vi "Count Up Down.vi"(6 "load":bool, 7 "reset":bool, 8 "error in":errorcluster, 9 "preset value":u32=10, 10 "count down":bool, 11 "count up":bool) -> (0 "error out":errorcluster, 1 "counter value":u32, 2 "count down done":bool, 3 "count up done":bool)   [LabVIEW 2020, in "NI_FunctionBlock Libraries.lvlib"]
uses:
  <vilib>/functionblocks/NI_FunctionBlock Libraries.lvlib
  <vilib>/ptbypt/NI_PtbyPt.lvlib
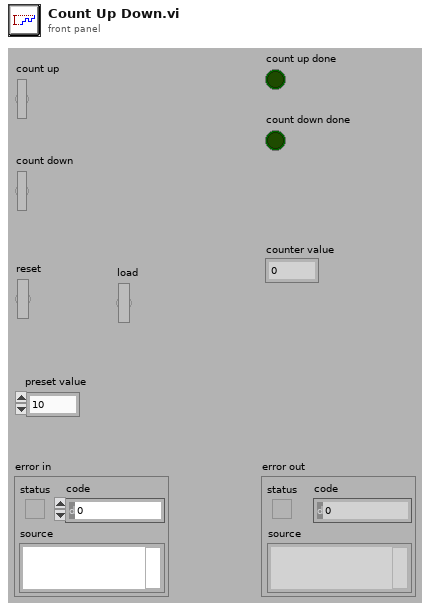
[diagram p1: front panel]
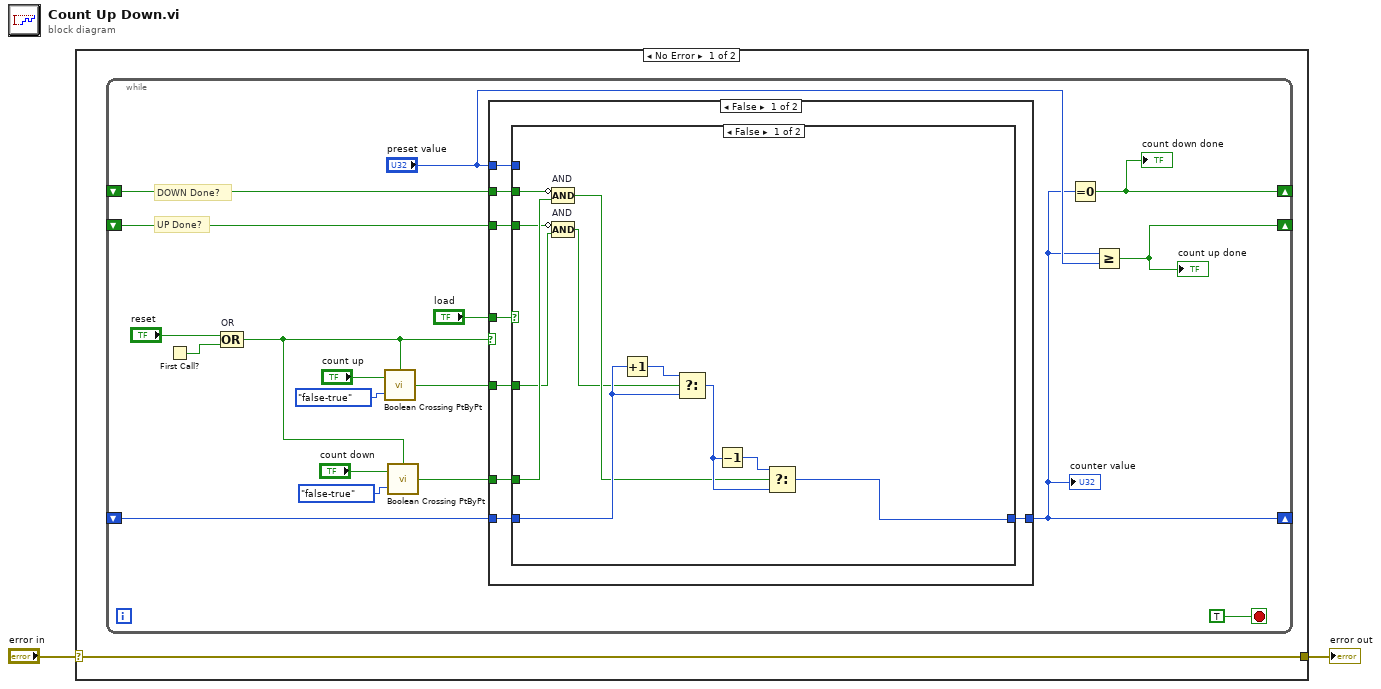
[diagram p0: block diagram]
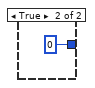
[diagram p3: hidden frame]
diagram:
  n1 = case shown="No Error" "error in" {
    selector: "error in" -> [w3 w43]
    tunnel: [w3 w43] -> w1
    frame No Error {
      n2 = while {
        shift-right: [w4] -> _
        shift-left: _ -> [w13]
        shift-right: [w5] -> _
        shift-left: _ -> [w11]
        shift-right: [w6] -> _
        shift-left: _ -> [w9]
        stop <- TRUE stop-if-true
        # "DOWN Done?"
        # "UP Done?"
        n3 = First Call?() -> (First Call?: T/F=w20:bool)
        n4 = Compound Arithmetic op=OR "OR"("reset", w20) -> (w14:bool)
        n5 = call <vilib>:"Boolean Crossing PtByPt.vi"("initialize"=w14, "direction"=enum16{"either", "false-true", "true-false"}."false-true", "input"="count up") -> ("crossing"=w8:bool)
        n6 = call <vilib>:"Boolean Crossing PtByPt.vi"("initialize"=w14, "direction"=enum16{"either", "false-true", "true-false"}."false-true", "input"="count down") -> ("crossing"=w10:bool)
        n7 = case shown="False" w14 {
          tunnel: [w26 u32 0] -> w4
          tunnel: w13 -> [w28 _]
          tunnel: w8 -> [w29 _]
          tunnel: w10 -> [w27 _]
          tunnel: "load" -> [w25 _]
          tunnel: w11 -> [w24 _]
          tunnel: w9 -> [w23 _]
          tunnel: "preset value" -> [w22 _]
          frame False {
            n8 = case shown="False" w25 {
              tunnel: w29 -> [w31 _]
              tunnel: w28 -> [w39 _]
              tunnel: w27 -> [w35 _]
              tunnel: [w30 w41] -> w26
              tunnel: w24 -> [w36 _]
              tunnel: w23 -> [w33 _]
              tunnel: w22 -> [_ w41]
              frame False {
                n9 = Compound Arithmetic op=AND "AND"(invert w36, w35) -> (w34:bool)
                n10 = Compound Arithmetic op=AND "AND"(invert w33, w31) -> (w32:bool)
                n11 = Increment(x=w39) -> (x+1=w40:u32)
                n12 = Select(t=w40, s=w32, f=w39) -> (s? t:f=w37:u32)
                n13 = Decrement(x=w37) -> (x-1=w38:u32)
                n14 = Select(t=w38, s=w34, f=w37) -> (s? t:f=w30:u32)
              }
              frame True {
              }
            }
          }
          frame True {
          }
        }
        "counter value" <- w4
        n15 = Equal To 0?(x=w4) -> (x = 0?=w5:bool)
        "count down done" <- w5
        n16 = Greater Or Equal?(x=w4, y="preset value") -> (x >= y?=w6:bool)
        "count up done" <- w6
      }
    }
    frame Error {
    }
  }
  "error out" <- w1
